vi "Magnetic Field.vi"(8 "error in (no error)":errorcluster, 10 "Power Supply in":refnum<class "Power Supply.lvclass">, 11 "Magnetic Field.lvclass in":refnum<class "Magnetic Field Oxford.lvclass">) -> (0 "error out":errorcluster, 3 "Magnetic Field.lvclass out":refnum<class "Magnetic Field Oxford.lvclass">)   [LabVIEW 2023, in "Magnetic Field Oxford.lvclass"]
uses:
  Magnetic Field Oxford.lvclass
  C:/LabVIEW-programs/Scanners/Scanner/Scanner.lvclass
  Instruments/Oxford Magnet/Power Supply/Power Supply.lvclass
  C:/LabVIEW-programs/Instruments/Utility Classes/Scannable/Scannable.lvclass
  Scanner/Scanner.lvclass
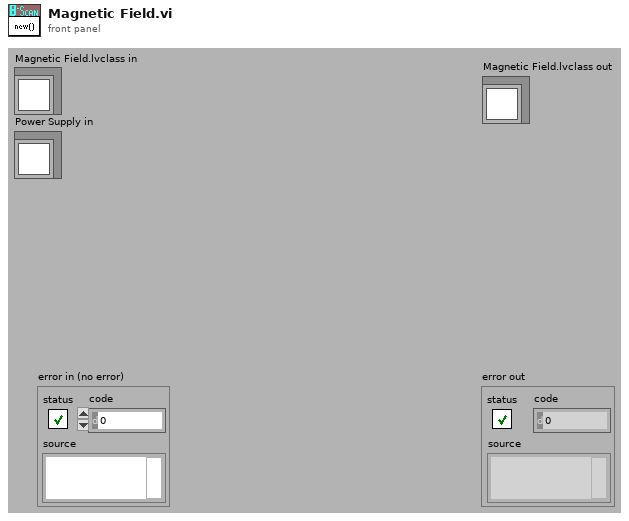
[diagram p1: front panel]
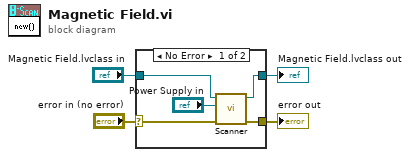
[diagram p0: block diagram]
diagram:
  n1 = case shown="No Error" "error in (no error)" {
    selector: "error in (no error)" -> [w9 w10]
    tunnel: [w8 w10] -> w3
    tunnel: [w6 w11] -> w1
    tunnel: "Magnetic Field.lvclass in" -> [w7 w11]
    frame No Error {
      n2 = call "Scanner.vi"("error in (no error)"=w9, "Scannable"="Power Supply in", "Scanner.lvclass in"=w7) -> ("error out"=w8:errorcluster, "Scanner.lvclass out"=w6:refnum<class "Magnetic Field Oxford.lvclass">)  [unwired: 1 in, 6 out]
    }
    frame Error {
    }
  }
  "error out" <- w3
  "Magnetic Field.lvclass out" <- w1
